vi "WriteDigitalOutput.vi"(8 "error in (no error)":errorcluster, 9 "Tristate":bool, 10 "data":bool, 11 "TesteractHAL_DigitalOutput_NIDAQmx In":refnum<class "TesteractHAL_DigitalOutput_NIDAQmx.lvclass">) -> (0 "error out":errorcluster, 3 "TesteractHAL_DigitalOutput_NIDAQmx Out":refnum<class "TesteractHAL_DigitalOutput_NIDAQmx.lvclass">)   [LabVIEW 2017, in "TesteractHAL_DigitalOutput_NIDAQmx.lvlib" / "TesteractHAL_DigitalOutput_NIDAQmx.lvclass"]
doc: "Writes a boolean to a single digital line."
uses:
  TesteractHAL_DigitalOutput_NIDAQmx.lvclass
  TesteractHAL_DigitalOutput_NIDAQmx.lvclass/TesteractHAL_DigitalOutput_NIDAQmx.ctl
  <vilib>/DAQmx/write.llb/DAQmx Write (Digital Bool 1Line 1Point).vi
  <vilib>/DAQmx/miscellaneous.llb/DAQmx Fill In Error Info.vi
  <resource>/objmgr/daqmx.rc
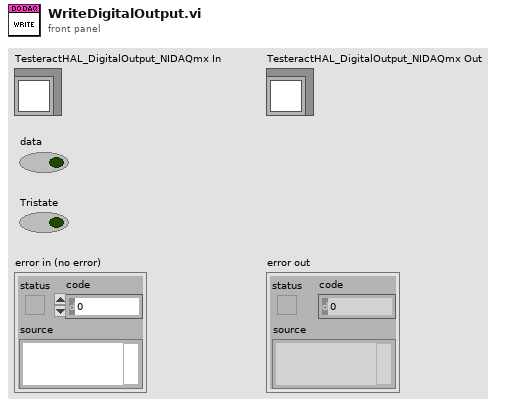
[diagram p1: front panel]
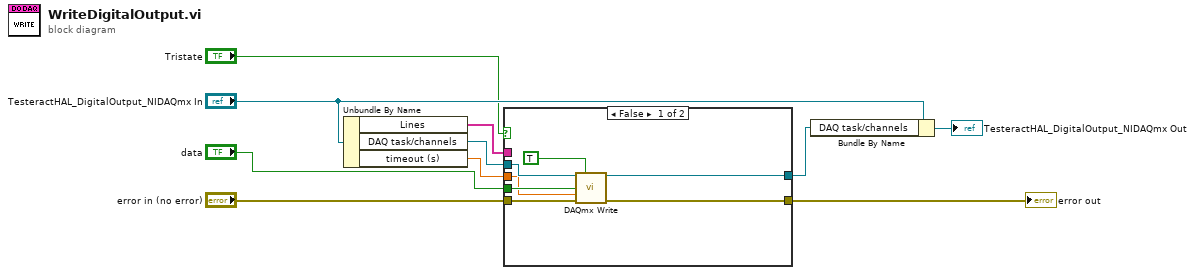
[diagram p0: block diagram]
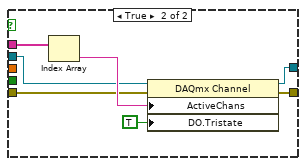
[diagram p2: hidden frame]
diagram:
  n1 = Unbundle By Name("TesteractHAL_DigitalOutput_NIDAQmx In") -> ("Lines"=w1:string[], "DAQ task/channels"=w10:refnum<k21>, "timeout (s)"=w3:dbl)
  n2 = case shown="False" "Tristate" {
    tunnel: w10 -> [w16 w22]
    tunnel: [w15 w20] -> w9
    tunnel: "data" -> [w14 _]
    tunnel: "error in (no error)" -> [w13 w21]
    tunnel: [w12 w19] -> w6
    tunnel: w3 -> [w11 _]
    tunnel: w1 -> [_ w24]
    frame False {
      n3 = call-poly <vilib>:"DAQmx Write.vi"("task/channels in"=w16, "auto start"=TRUE, "data"=w14, "timeout"=w11, "error in"=w13) -> ("task out"=w15:refnum<k21>, "error out"=w12:errorcluster)  [unwired: 8 in, 1 out]
    }
    frame True {
      n4 = Index Array(array=w24) -> (element=w23:string)  [unwired: 1 in]
      n5 = property class="DAQmx Channel"(reference=w22, error in=w21, "ActiveChans"=w23, "DO.Tristate"=TRUE) -> (reference out=w20:refnum<k21>, error out=w19:errorcluster)
    }
  }
  "error out" <- w6
  n6 = Bundle By Name(cluster="TesteractHAL_DigitalOutput_NIDAQmx In", "DAQ task/channels"=w9) -> (→"TesteractHAL_DigitalOutput_NIDAQmx Out":refnum<class "TesteractHAL_DigitalOutput_NIDAQmx.lvclass">)
